vi "Sample_SimpleBoolRead.vi"() -> ()   [LabVIEW 2022 SP3, in "ADS_Library.lvlib"]
uses:
  ADS_Library.lvlib
panel:
  out "error out":errorcluster
  out "Boolean":bool
  out "Read status?":bool
  out "RData":variant
  in  "String":string
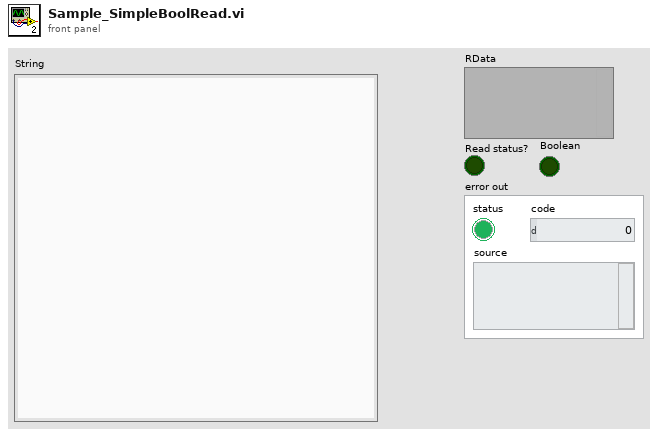
[diagram p1: front panel]
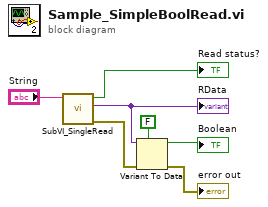
[diagram p0: block diagram]
diagram:
  n1 = call "SubVI_SingleRead.vi"("String"="String") -> ("error out"=w4:errorcluster, "RData"=w5:variant, "Read status?"=→"Read status?":bool)  [unwired: 7 in]
  "RData" <- w5
  n2 = Variant To Data(error in=w4, type=FALSE, Variant=w5) -> (data=→"Boolean":bool, error out=→"error out":errorcluster)
